vi "SW_Get_temporary_save_path.vi"(0 "Temporary file name prefix":string="TrackTemp") -> (2 "date/time string":string, 3 "Temporary file output path":path, 4 "Temporary archive output path":path, 5 "Name in zip":path)   [LabVIEW 2018, in "Tracker.lvlib"]
uses:
  <vilib>/Utility/sysdir.llb/System Directory Type.ctl
  Tracker.lvlib
panel:
  in  "error in (no error)":errorcluster
  out "error out":errorcluster
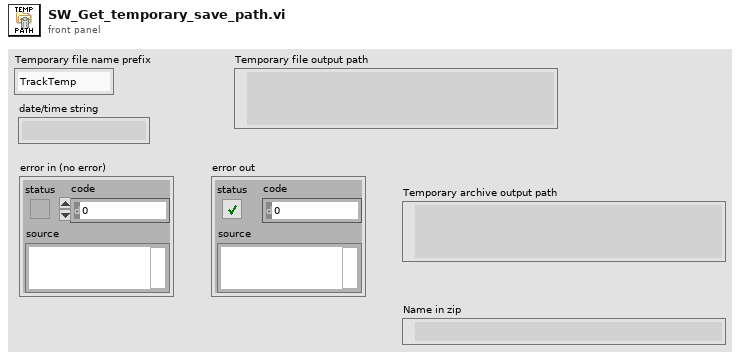
[diagram p1: front panel]
types:
  T1 = typedef "System Directory Type.ctl" = i32
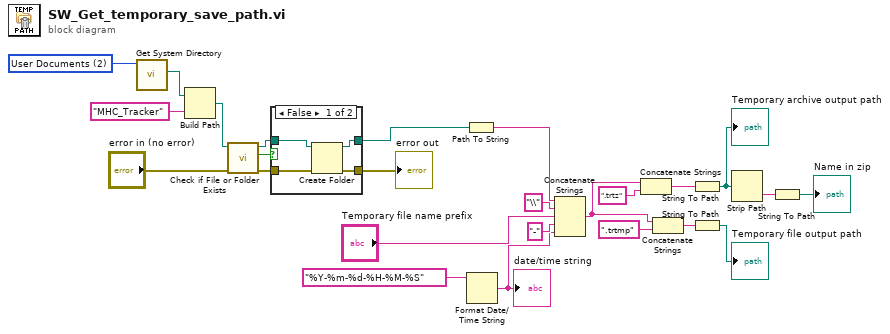
[diagram p0: block diagram]
diagram:
  w18 = T1 2 items=["User Home"=0, "User Desktop"=1, "User Documents"=2, "User Application Data"=3, "User Preferences"=4, "User Temporary"=5, "Public Documents"=6, "Public Application Data"=7, "Public Preferences"=8, "Public Cache"=13, "System Core Libraries"=9, "System Installed Libraries"=10, "Application Files"=11, "Boot Volume Root"=12] ("system directory type")
  n1 = call <vilib>:"Get System Directory.vi"("system directory type"=w18) -> ("system directory"=w16:path)  [unwired: 10 in]
  n2 = Build Path(base path=w16, name or relative path="MHC_Tracker" ("string")) -> (appended path=w15:path)
  n3 = call <vilib>:"Check if File or Folder Exists.vi"("error in (no error)"="error in (no error)", "path"=w15) -> ("error out"=w12:errorcluster, "file or folder exists?"=w14:bool, "dup path"=w13:path)  [unwired: 7 in]
  n4 = case shown="False" w14 {
    tunnel: w13 -> [w28 w31]
    tunnel: w12 -> [w29 w30]
    tunnel: [w27 w31] -> w11
    tunnel: [w26 w30] -> w10
    frame False {
      n5 = Create Folder(path (use dialog)=w28, error in=w29) -> (created path=w27:path, error out=w26:errorcluster)  [unwired: 1 in, 1 out]
    }
    frame True {
    }
  }
  "error out" <- w10
  n6 = Path To String(path=w11) -> (string=w25:string)
  n7 = Format Date/Time String(time format string (%c)="%Y-%m-%d-%H-%M-%S") -> (date/time string=w19:string)  [unwired: 2 in]
  "date/time string" <- w19
  n8 = Concatenate Strings(w25, "\\" ("string"), "Temporary file name prefix", "-" ("string"), w19) -> (w6:string)
  n9 = Concatenate Strings(w6, ".trtz" ("string")) -> (w4:string)
  n10 = Concatenate Strings(w6, ".trtmp" ("string")) -> (w7:string)
  n11 = String To Path(string=w4) -> (path=w3:path)
  "Temporary archive output path" <- w3
  n12 = String To Path(string=w7) -> (path=→"Temporary file output path":path)
  n13 = Strip Path(path=w3) -> (name=w2:string)  [unwired: 1 out]
  n14 = String To Path(string=w2) -> (path=→"Name in zip":path)
